vi "Record Joysticks.vi"(7 "Auto Name":string, 8 "error in (no error)":errorcluster, 9 "Turn X joystick":dbl, 10 "Speed Y Joystick":dbl, 11 "Function":enum16{"Start Log", "Log Data", "Stop Log"}(ring)=enum."Stop Log") -> (0 "error out":errorcluster={"status"=TRUE, "code"=1430, "source"="Move in DATA LOGGER.VI->Test Data Logger.vi<APPEND>\n<Not A Path>"})   [LabVIEW 2019]
panel:
  out "Filename":path
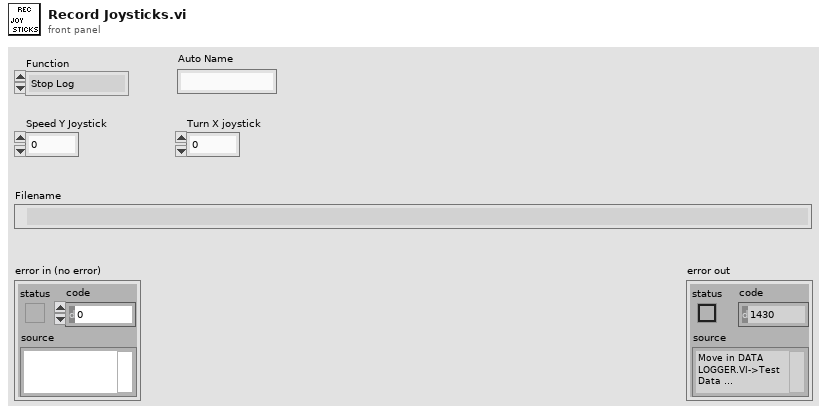
[diagram p1: front panel]
types:
  T1 = enum16{"open", "replace", "create", "open or create", "replace or create", "replace or create with confirmation"}
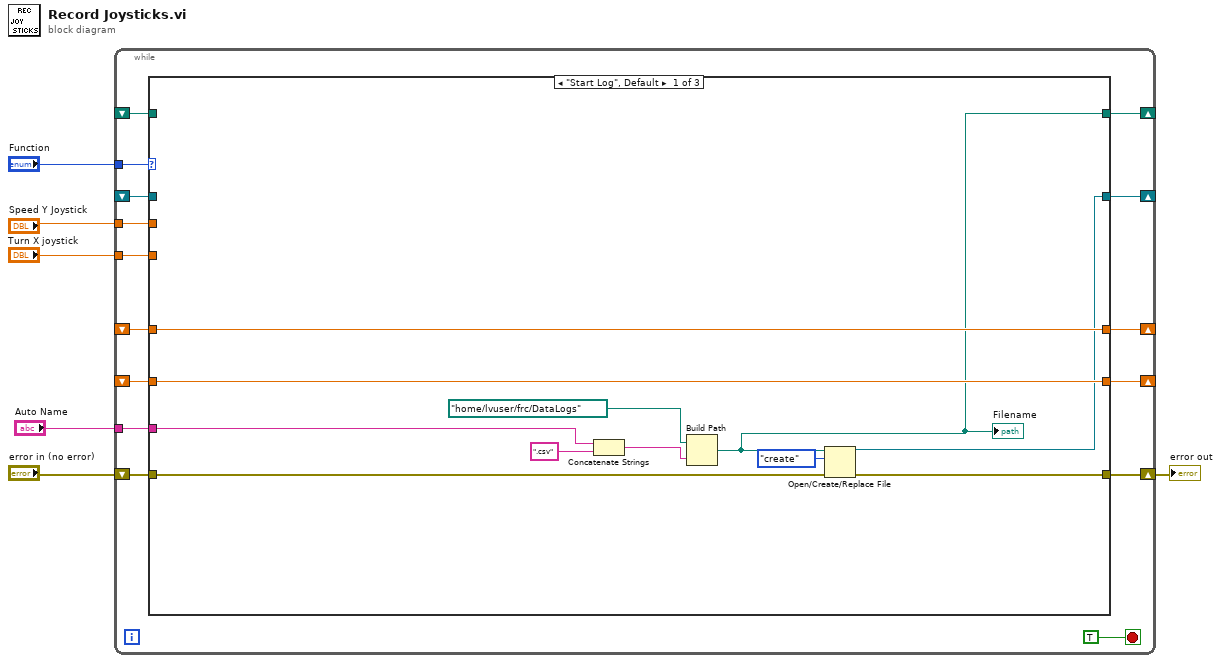
[diagram p0: block diagram]
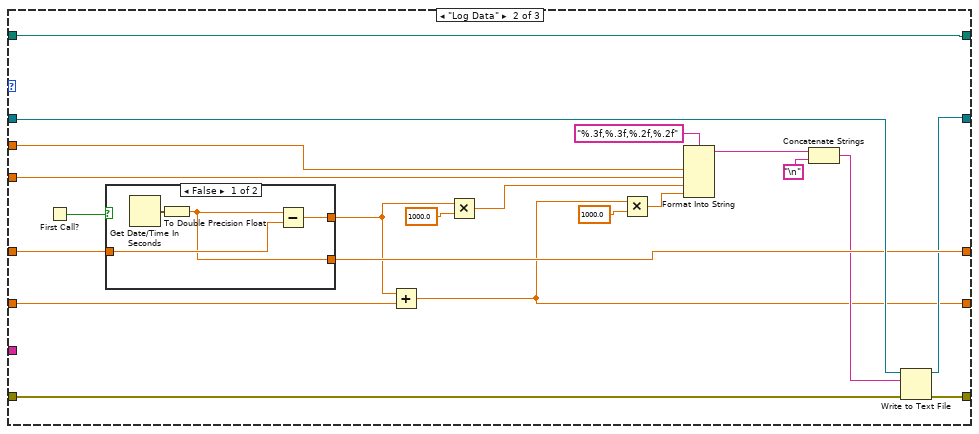
[diagram p2: hidden frame]
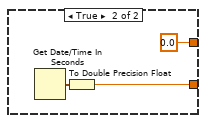
[diagram p3: hidden frame]
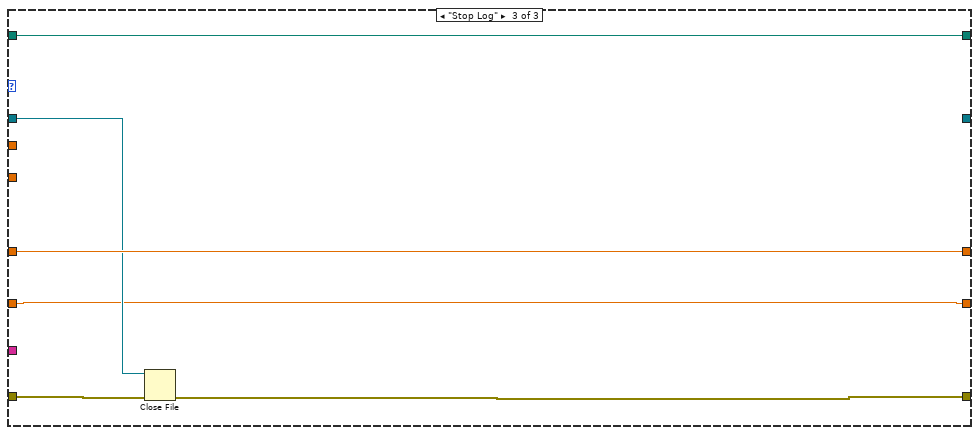
[diagram p4: hidden frame]
diagram:
  n1 = while {
    shift-right: [w20] -> w3
    shift-left: "error in (no error)" -> [w21]
    shift-right: [w19] -> _
    shift-left: _ -> [w18]
    tunnel: "Speed Y Joystick" -> [w17]
    tunnel: "Turn X joystick" -> [w16]
    tunnel: "Function" -> [w14]
    shift-right: [w13] -> _
    shift-left: _ -> [w12]
    shift-right: [w11] -> _
    shift-left: _ -> [w10]
    shift-right: [w9] -> _
    shift-left: _ -> [w8]
    tunnel: "Auto Name" -> [w7]
    stop <- TRUE stop-if-true
    n2 = case shown="\"Start Log\", Default" w14 {
      tunnel: [w22 w53 w61] -> w20
      tunnel: w21 -> [w32 w40 w65]
      tunnel: [w23 w50 _] -> w19
      tunnel: w18 -> [_ w52 w64]
      tunnel: w17 -> [_ w43 _]
      tunnel: w16 -> [_ w42 _]
      tunnel: [w31 w51 w66] -> w13
      tunnel: w12 -> [w31 w45 w66]
      tunnel: [w24 w49 w63] -> w11
      tunnel: w10 -> [_ w49 w63]
      tunnel: [w30 w34 w62] -> w9
      tunnel: w8 -> [w30 w38 w62]
      tunnel: w7 -> [w27 _ _]
      frame "Start Log", Default {
        n3 = Concatenate Strings(w27, ".csv" ("string")) -> (w25:string)
        n4 = Build Path(base path=path "/home/lvuser/frc/DataLogs", name or relative path=w25) -> (appended path=w24:path)
        "Filename" <- w24
        n5 = Open/Create/Replace File(file path (use dialog)=w24, error in=w32, operation (0:open)=T1."create") -> (refnum out=w23:refnum<file>, error out=w22:errorcluster)  [unwired: 3 in, 1 out]
      }
      frame "Log Data" {
        n6 = First Call?() -> (First Call?: T/F=w46:bool)
        n7 = case shown="False" w46 {
          tunnel: [w55 0.0] -> w39
          tunnel: [w54 w58] -> w51
          tunnel: w45 -> [w56 _]
          frame False {
            n8 = Get Date/Time In Seconds() -> (seconds since 1Jan1904=w57:timestamp)
            n9 = To Double Precision Float(number=w57) -> (double precision float=w54:dbl)
            n10 = Subtract(x=w54, y=w56) -> (x-y=w55:dbl)
          }
          frame True {
            n11 = Get Date/Time In Seconds() -> (seconds since 1Jan1904=w59:timestamp)
            n12 = To Double Precision Float(number=w59) -> (double precision float=w58:dbl)
          }
        }
        n13 = Add(x=w39, y=w38) -> (x+y=w34:dbl)
        n14 = Multiply(x=w39, y=1000.0) -> (x*y=w37:dbl)
        n15 = Multiply(x=w34, y=1000.0) -> (x*y=w33:dbl)
        n16 = Format Into String(format string="%.3f,%.3f,%.2f,%.2f", w43, w42, w37, w33) -> (resulting string=w41:string)  [unwired: 2 in, 1 out]
        n17 = Concatenate Strings(w41, "\n") -> (w47:string)
        n18 = Write to Text File(file (use dialog)=w52, text=w47, error in=w40) -> (refnum out=w50:refnum<file>, error out=w53:errorcluster)  [unwired: 1 in, 1 out]
      }
      frame "Stop Log" {
        n19 = Close File(refnum=w64, error in=w65) -> (error out=w61:errorcluster)  [unwired: 1 out]
      }
    }
  }
  "error out" <- w3
